vi "timdelay.vi"(8 "error in (no error)":errorcluster caption="错误输入（无错误）", 10 "等待时间（毫秒）":u32=100) -> (0 "error in (no error) 2":errorcluster caption="错误输入（无错误）")   [LabVIEW 2014]
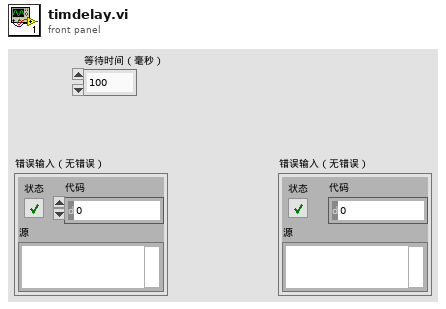
[diagram p1: front panel]
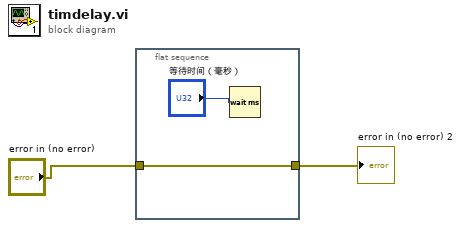
[diagram p0: block diagram]
diagram:
  n1 = flat-sequence {
    tunnel: "error in (no error)" -> [w3]
    tunnel: [w3] -> w1
    frame #0 {
      n2 = Wait (ms)(milliseconds to wait="等待时间（毫秒）") -> ()  [unwired: 1 out]
    }
  }
  "error in (no error) 2" <- w1
